vi "Execute.vi"(8 "error in (no error)":errorcluster, 9 "Consumer Queues in":T1, 10 "DAC Process Command in":refnum<class "Init DAC Process.lvclass">, 11 "DAC Process Data in":T2) -> (0 "error out":errorcluster, 1 "Consumer Queues out":T1, 2 "Stop?":bool, 3 "DAC Process Data out":T2)   [LabVIEW 2019, in "DAC Process.lvlib" / "Init DAC Process.lvclass"]
uses:
  Init DAC Process.lvclass
  DAC Process Data.ctl
  Generic Test Stand/Generic Test Stand.lvclass
  TS Framework/ExeLogging/DAC Logger/DAC Logger.lvclass
  DAC State.ctl
  TS Framework/Consumer Queues.ctl
  UI Process/Generic UI Command/Generic UI Process Command.lvclass
  Generic DAC Command/Generic DAC Process Command.lvclass
  Trig Process/Generic Trig Command/Generic Trig Process Command.lvclass
  Setup DAC Test Stand/Setup DAC Test Stand.lvclass
  Init DAC Process.lvclass/Init DAC Process.ctl
  Generic Test Stand/Generic Test Stand.lvclass/Generic Test Stand.ctl
  Setup DAC Test Stand/Setup DAC Test Stand.lvclass/Setup DAC Test Stand.ctl
  DAC Process.lvlib
  TS Framework/TS Framework.lvlib
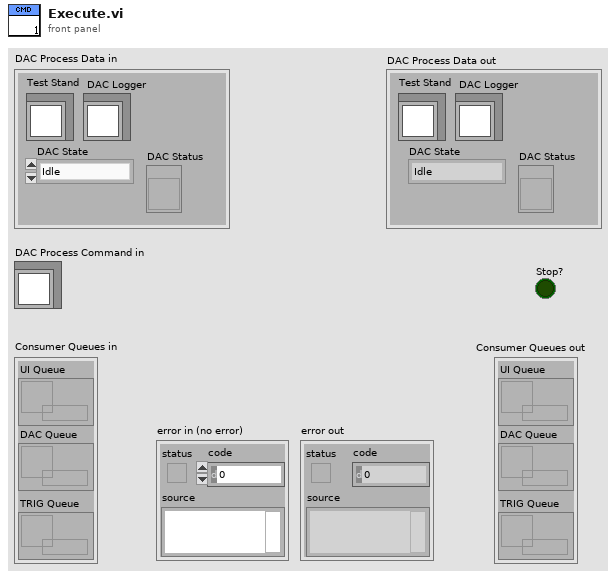
[diagram p1: front panel]
types:
  T1 = typedef "TS Framework.lvlib/Consumer Queues.ctl" = cluster{"UI Queue":refnum<queue>, "DAC Queue":refnum<queue>, "TRIG Queue":refnum<queue>}
  T2 = typedef "DAC Process.lvlib/DAC Process Data.ctl" = cluster{"Test Stand":refnum<class "Generic Test Stand.lvclass">, " DAC Logger":refnum<class "DAC Logger.lvclass">, "DAC State":T3, "DAC Status":refnum<vi>}
  T3 = typedef "DAC Process.lvlib/DAC State.ctl" = enum16{"Idle", "Acquiring"}
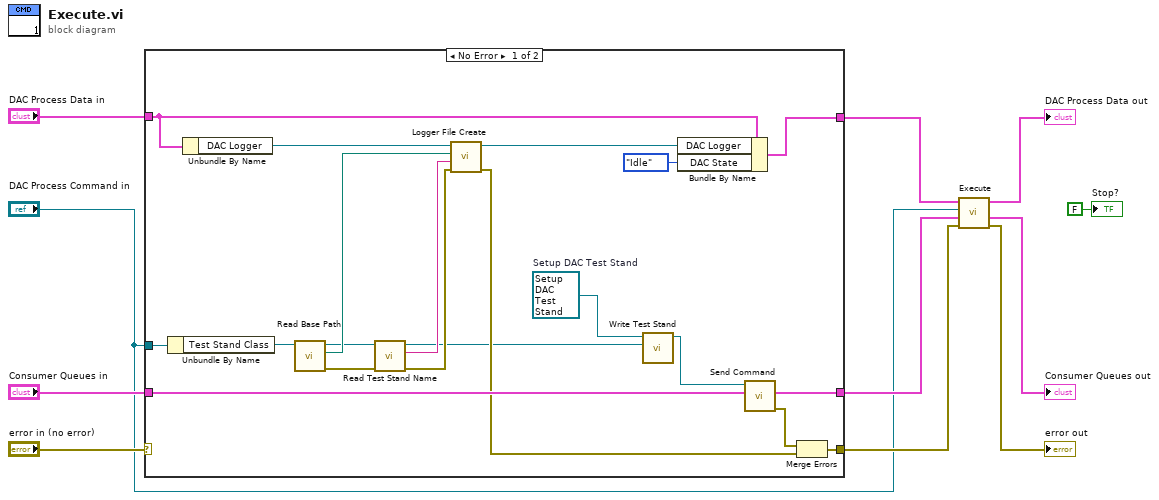
[diagram p0: block diagram]
diagram:
  n1 = case shown="No Error" "error in (no error)" {
    selector: "error in (no error)" -> [_ w33]
    tunnel: "DAC Process Command in" -> [w24 _]
    tunnel: "Consumer Queues in" -> [w22 w32]
    tunnel: [w21 w32] -> w4
    tunnel: "DAC Process Data in" -> [w28 w34]
    tunnel: [w26 w34] -> w5
    tunnel: [w20 w33] -> w3
    frame No Error {
      w14 = refnum<class "Setup DAC Test Stand.lvclass"> refnum  # Setup DAC Test Stand
      n2 = Unbundle By Name(w24) -> ("Test Stand Class"=w27:refnum<class "Generic Test Stand.lvclass">)
      n3 = Unbundle By Name(w28) -> ("DAC Logger"=w31:refnum<class "DAC Logger.lvclass">)
      n4 = call "Read Base Path.vi"("Generic Test Stand in"=w27) -> ("error out"=w17:errorcluster, "Base Path"=w30:path, "Generic Test Stand out"=w25:refnum<class "Generic Test Stand.lvclass">)  [unwired: 8 in]
      n5 = call "Read Test Stand Name.vi"("error in (no error)"=w17, "Generic Test Stand in"=w25) -> ("error out"=w16:errorcluster, "Test Stand Name"=w23:string, "Generic Test Stand out"=w15:refnum<class "Generic Test Stand.lvclass">)  [unwired: 7 in]
      n6 = call-dynamic "Logger File Create.vi"("error in"=w16, "Test Stand Name"=w23, "Project Base Path"=w30, "DAC Logger in"=w31) -> ("error out"=w19:errorcluster, "DAC Logger out"=w29:refnum<class "DAC Logger.lvclass">)  [unwired: 6 in]
      n7 = call "Write Test Stand.vi"("Generic Test Stand.lvclass"=w15, "Setup DAC Test Stand in"=w14) -> ("Setup DAC Test Stand out"=w13:refnum<class "Setup DAC Test Stand.lvclass">)  [unwired: 8 in, 1 out]
      n8 = Bundle By Name(cluster=w28, "DAC Logger"=w29, "DAC State"=DAC_State."Idle") -> (w26:T2)
      n9 = call-dynamic "Send Command.vi"("Consumer Queues in"=w22, "DAC Process Command"=w13) -> ("error out"=w18:errorcluster, "Consumer Queues out"=w21:T1)  [unwired: 8 in]
      n10 = Merge Errors(w18, w19) -> (w20:errorcluster)
    }
    frame Error {
    }
  }
  n11 = call-parent "Execute.vi"("error in"=w3, "Consumer Queues in"=w4, "DAC Process Command in"="DAC Process Command in", "DAC Process Data in"=w5) -> ("error out"=→"error out":errorcluster, "Consumer Queues out"=→"Consumer Queues out":T1, "DAC Process Data out"=→"DAC Process Data out":T2)  [unwired: 4 in, 1 out]
  "Stop?" <- FALSE ("Stop?")
